vi "00 - Simplest VI.vi"() -> ()   [LabVIEW 2025]
panel:
  in  "INACTIVE by default":bool
  out "Waveform Chart":dbl(graph)
  in  "Vertical Pointer Slide":dbl(slide) scale=0.0..10.0
  # "To experiment with configuration\nClick the above button that looks like this"
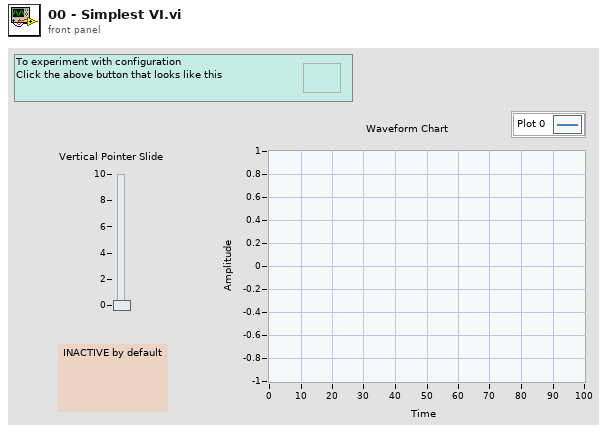
[diagram p1: front panel]
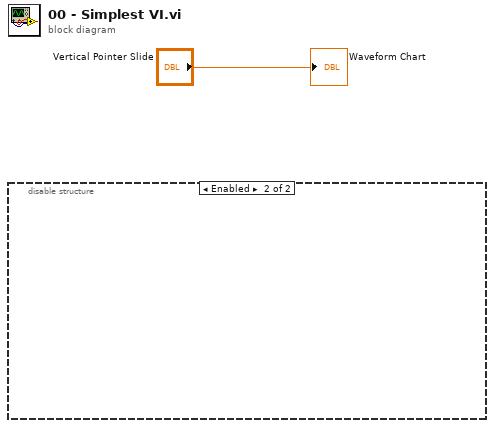
[diagram p0: block diagram]
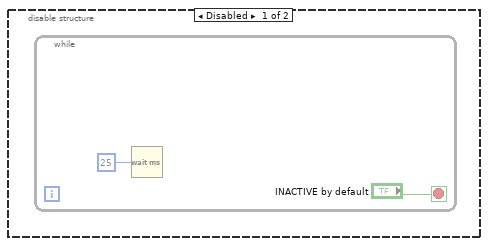
[diagram p2: hidden frame]
diagram:
  n1 = disable-structure shown="Enabled" {
    frame Disabled {
      n2 = while {
        stop <- "INACTIVE by default" stop-if-true
        n3 = Wait (ms)(milliseconds to wait=u32 25) -> ()  [unwired: 1 out]
      }
    }
    frame Enabled {
    }
  }
  "Waveform Chart" <- "Vertical Pointer Slide"
